vi "Write modulator.clock delay.vi"(8 "error in (no error)":errorcluster, 10 "modulator.clock delay":fxp<+,4,4>, 11 "rqcBob in":refnum<class "rqcBob.lvclass">) -> (0 "error out":errorcluster, 3 "rqcBob out":refnum<class "rqcBob.lvclass">)   [LabVIEW 2018, in "rqcBob.lvclass"]
uses:
  rqcBob.lvclass
  Custom Controls/rqcBob Main FPGA interface.ctl
  rqcBob.lvclass/rqcBob.ctl
  <vilib>/Utility/error.llb/Error Cluster From Error Code.vi
  <vilib>/rvi/errors/niLvFpgaAdjustHostInterfaceError.vi
  <vilib>/rvi/interface/nirviReadWriteControl/nirviReadWriteControl.xnode
  NiFpgaLv.dll
  <vilib>/rvi/interface/Simulation/niFpgaSimulationCallBeginRW.vi
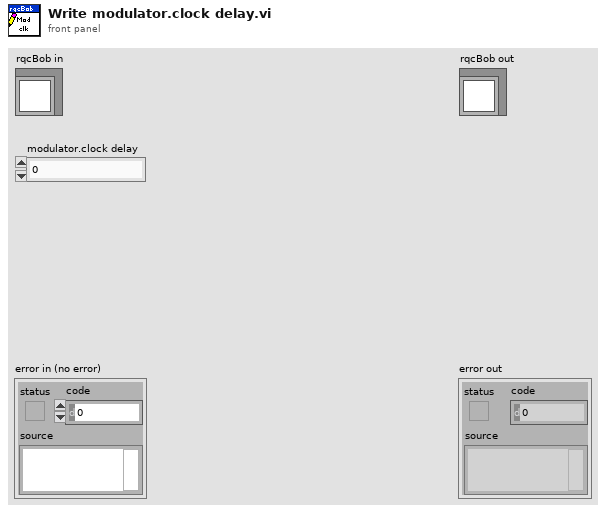
[diagram p1: front panel]
types:
  T1 = typedef "rqcBob.lvclass/rqcBob Main FPGA interface.ctl" = refnum<k20>
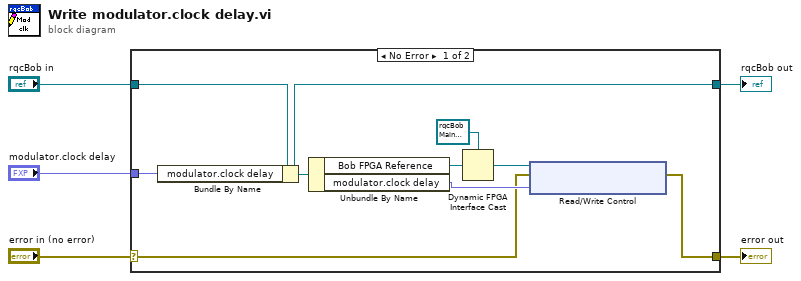
[diagram p0: block diagram]
diagram:
  n1 = case shown="No Error" "error in (no error)" {
    selector: "error in (no error)" -> [w7 w15]
    tunnel: [w6 w15] -> w4
    tunnel: [w9 w16] -> w2
    tunnel: "rqcBob in" -> [w14 w16]
    tunnel: "modulator.clock delay" -> [w13 _]
    frame No Error {
      n2 = Bundle By Name(cluster=w14, "modulator.clock delay"=w13) -> (w9:refnum<class "rqcBob.lvclass">)
      n3 = Unbundle By Name(w9) -> ("Bob FPGA Reference"=w12:refnum<k20>, "modulator.clock delay"=w10:fxp<+,4,4>)
      n4 = Dynamic FPGA Interface Cast(Session In=T1 refnum ("Bob main FPGA interface"), Type=w12) -> (Session Out=w11:T1)
      n5 = xnode "Read/Write Control"("FPGA VI Reference In"=w11, "error in"=w7, "modulator.clock delay"=w10) -> ("error out"=w6:errorcluster)  [unwired: 1 out]
    }
    frame Error {
    }
  }
  "error out" <- w4
  "rqcBob out" <- w2
